vi "STO_Recover.vi"() -> ()   [LabVIEW 2016]
uses:
  <vilib>/Stratom, Inc/X-CAN for myRIO (API)/X-CAN Class/Type Definitions/CANFrame.ctl
  <vilib>/Stratom, Inc/X-Modules for myRIO/Type Defs/MXPChannel.ctl
  <vilib>/Stratom, Inc/X-CAN for myRIO (API)/X-CAN Class/Type Definitions/CAN_Speed.ctl
  <vilib>/myRIO/Common/Instrument Driver Framework/myRIO v1.0/UART/vis/myRIO v1.0 Close UART.vi
  <vilib>/myRIO/Common/Instrument Driver Framework/Utilities/vis/FPGA Ref Manager.vi
  <vilib>/myRIO/Common/Instrument Driver Framework/myRIO v1.0/myRIO v1.0 Reset FPGA.vi
  <vilib>/myRIO/Common/Instrument Driver Framework/myRIO v1.0/IRQ/vis/myRIO v1.0 IRQ Info FGV.vi
  <vilib>/myRIO/Common/Instrument Driver Framework/myRIO v1.0/IRQ/vis/myRIO v1.0 Timer IRQ Info FGV.vi
  <vilib>/myRIO/Common/Instrument Driver Framework/myRIO v1.0/IRQ/vis/myRIO v1.0 ISR Agent.vi
  <vilib>/Stratom, Inc/X-CAN for myRIO (API)/X-CAN Class/X-CAN.lvclass
  <vilib>/myRIO/Instrument Drivers/Utilities/Utilities.lvlib
panel:
  out "Enable_Mtr1":T1 {"payload" format="%x"; "timestamp" format="%<%I:%M:%S%8u %p\n%x>T"; "identifier" format="%x"}
  out "CAN Frame 8":T1 {"payload" format="%x"; "timestamp" format="%<%I:%M:%S%8u %p\n%x>T"; "identifier" format="%x"}
  out "Enable_Mtr2":T1 {"payload" format="%x"; "timestamp" format="%<%I:%M:%S%8u %p\n%x>T"; "identifier" format="%x"}
  out "CAN Frame 6":T1 {"payload" format="%x"; "timestamp" format="%<%I:%M:%S%8u %p\n%x>T"; "identifier" format="%x"}
  in  "Motor1(P)_______Motor2(D)":bool
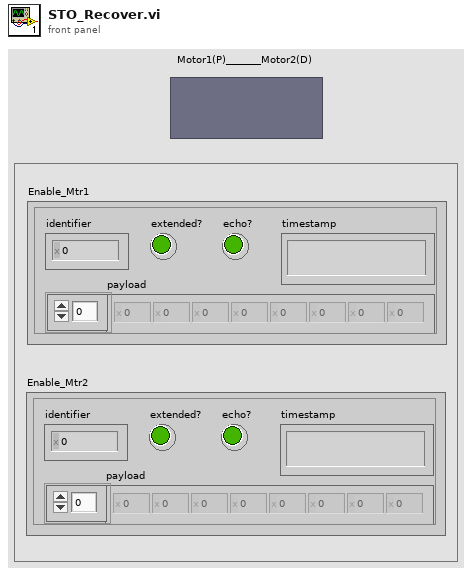
[diagram p1: front panel]
types:
  T1 = typedef "X-CAN.lvclass/CANFrame.ctl" = cluster{"identifier":u32, "extended?":bool, "echo?":bool, "payload":u8[], "timestamp":timestamp}
  T2 = typedef "X-CAN.lvclass/CAN_Speed.ctl" = u8
  T3 = typedef "MXPChannel.ctl" = enum16{"A/MXP", "B/MXP"}
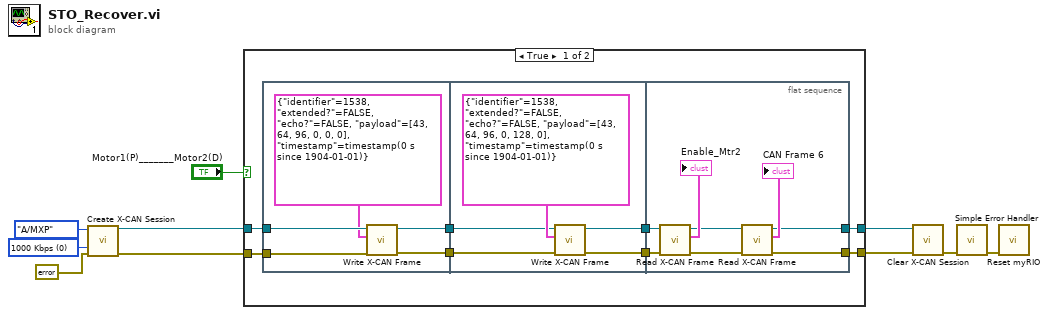
[diagram p0: block diagram]
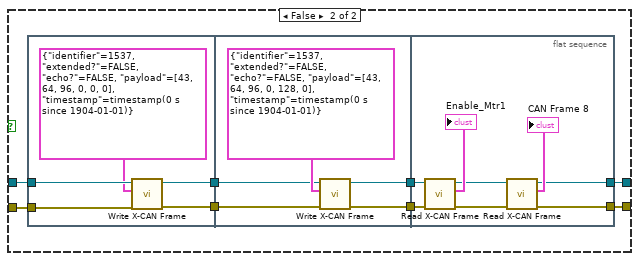
[diagram p2: hidden frame]
diagram:
  w7 = T2 0 items=["125 Kbps"=7, "250 Kbps"=3, "500 Kbps"=1, "1000 Kbps"=0, "95.238 Kbps"=6] ("CAN Speed [Kbps]")
  n1 = call <vilib>:"Create X-CAN Session.vi"("error in (no error)"=errorcluster {"status"=FALSE, "code"=0, "source"=""}, "CAN Speed [Kbps]"=w7, "MXP Channel"=MXPChannel."A/MXP") -> ("error out"=w5:errorcluster, "X-CAN Session out"=w4:refnum<class "X-CAN.lvclass">)  [unwired: 7 in]
  n2 = case shown="True" "Motor1(P)_______Motor2(D)" {
    tunnel: [w14 w40] -> w2
    tunnel: [w13 w39] -> w3
    tunnel: w5 -> [w12 w38]
    tunnel: w4 -> [w11 w37]
    frame True {
      n3 = flat-sequence {
        tunnel: w12 -> [w21]
        tunnel: w11 -> [w20]
        tunnel: [w23] -> w18
        tunnel: [w22] -> w17
        tunnel: w18 -> [w26]
        tunnel: w17 -> [w27]
        tunnel: [w25] -> w16
        tunnel: [w24] -> w15
        tunnel: [w29] -> w13
        tunnel: [w34] -> w14
        tunnel: w16 -> [w36]
        tunnel: w15 -> [w33]
        frame #0 {
          n4 = call <vilib>:"Write X-CAN Frame.vi"("error in"=w21, "CAN Frame"=T1 {"identifier"=1538, "extended?"=FALSE, "echo?"=FALSE, "payload"=[43, 64, 96, 0, 0, 0], "timestamp"=timestamp(0 s since 1904-01-01)}, "X-CAN Session in"=w20) -> ("error out"=w23:errorcluster, "X-CAN Session out"=w22:refnum<class "X-CAN.lvclass">)  [unwired: 7 in]
        }
        frame #1 {
          n5 = call <vilib>:"Write X-CAN Frame.vi"("error in"=w26, "CAN Frame"=T1 {"identifier"=1538, "extended?"=FALSE, "echo?"=FALSE, "payload"=[43, 64, 96, 0, 128, 0], "timestamp"=timestamp(0 s since 1904-01-01)}, "X-CAN Session in"=w27) -> ("error out"=w25:errorcluster, "X-CAN Session out"=w24:refnum<class "X-CAN.lvclass">)  [unwired: 7 in]
        }
        frame #2 {
          n6 = call <vilib>:"Read X-CAN Frame.vi"("error in"=w36, "X-CAN Session in"=w33) -> ("error out"=w35:errorcluster, "CAN Frame"=→"Enable_Mtr2":T1, "X-CAN Session out"=w30:refnum<class "X-CAN.lvclass">)  [unwired: 7 in]
          n7 = call <vilib>:"Read X-CAN Frame.vi"("error in"=w35, "X-CAN Session in"=w30) -> ("error out"=w34:errorcluster, "CAN Frame"=→"CAN Frame 6":T1, "X-CAN Session out"=w29:refnum<class "X-CAN.lvclass">)  [unwired: 7 in]
        }
      }
    }
    frame False {
      n8 = flat-sequence {
        tunnel: w38 -> [w47]
        tunnel: w37 -> [w46]
        tunnel: [w49] -> w44
        tunnel: [w48] -> w43
        tunnel: w44 -> [w52]
        tunnel: w43 -> [w53]
        tunnel: [w51] -> w42
        tunnel: [w50] -> w41
        tunnel: [w55] -> w39
        tunnel: [w60] -> w40
        tunnel: w42 -> [w62]
        tunnel: w41 -> [w59]
        frame #0 {
          n9 = call <vilib>:"Write X-CAN Frame.vi"("error in"=w47, "CAN Frame"=T1 {"identifier"=1537, "extended?"=FALSE, "echo?"=FALSE, "payload"=[43, 64, 96, 0, 0, 0], "timestamp"=timestamp(0 s since 1904-01-01)}, "X-CAN Session in"=w46) -> ("error out"=w49:errorcluster, "X-CAN Session out"=w48:refnum<class "X-CAN.lvclass">)  [unwired: 7 in]
        }
        frame #1 {
          n10 = call <vilib>:"Write X-CAN Frame.vi"("error in"=w52, "CAN Frame"=T1 {"identifier"=1537, "extended?"=FALSE, "echo?"=FALSE, "payload"=[43, 64, 96, 0, 128, 0], "timestamp"=timestamp(0 s since 1904-01-01)}, "X-CAN Session in"=w53) -> ("error out"=w51:errorcluster, "X-CAN Session out"=w50:refnum<class "X-CAN.lvclass">)  [unwired: 7 in]
        }
        frame #2 {
          n11 = call <vilib>:"Read X-CAN Frame.vi"("error in"=w62, "X-CAN Session in"=w59) -> ("error out"=w61:errorcluster, "CAN Frame"=→"Enable_Mtr1":T1, "X-CAN Session out"=w56:refnum<class "X-CAN.lvclass">)  [unwired: 7 in]
          n12 = call <vilib>:"Read X-CAN Frame.vi"("error in"=w61, "X-CAN Session in"=w56) -> ("error out"=w60:errorcluster, "CAN Frame"=→"CAN Frame 8":T1, "X-CAN Session out"=w55:refnum<class "X-CAN.lvclass">)  [unwired: 7 in]
        }
      }
    }
  }
  n13 = call <vilib>:"Clear X-CAN Session.vi"("error in (no error)"=w2, "X-CAN Session in"=w3) -> ("error out"=w10:errorcluster)  [unwired: 9 in]
  n14 = call <vilib>:"Simple Error Handler.vi"("error in (no error)"=w10) -> ("error out"=w9:errorcluster)  [unwired: 4 in, 4 out]
  n15 = call <vilib>:"Reset myRIO.vi"("error in (no error)"=w9) -> ()  [unwired: 10 in, 1 out]
